vi "初始化.vi"(0 "counter":tag="Dev2/ctr2", 5 "channel name":string="T1", 7 "low time":dbl=0.00026 format="%0.2e", 9 "high time":dbl=0.00024 format="%0.2e", 11 "error in":errorcluster caption="错误输入") -> (4 "task out":refnum<k21> caption="任务输出", 15 "error out":errorcluster caption="错误输出")   [LabVIEW 2020]
uses:
  <vilib>/DAQmx/create/channels.llb/DAQmx Create Channel (CO-Pulse Generation-Time).vi
  <vilib>/DAQmx/configure/timing.llb/DAQmx Timing (Implicit).vi
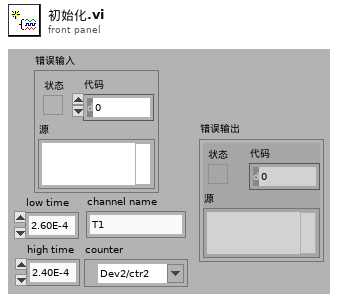
[diagram p1: front panel]
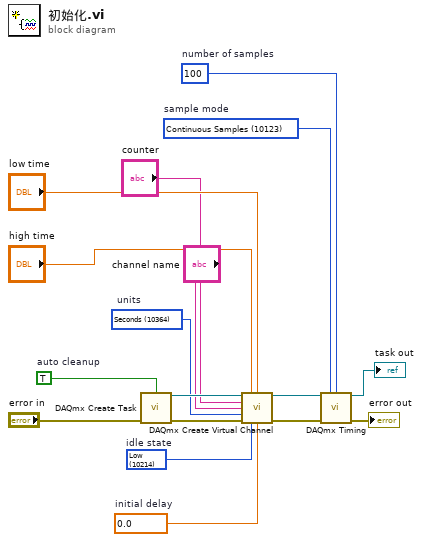
[diagram p0: block diagram]
diagram:
  w2 = 10123 items=["Finite Samples"=10178, "Continuous Samples"=10123, "Hardware Timed Single Point"=12522]  # sample mode
  w3 = 100  # number of samples
  w9 = 0.0  # initial delay
  w10 = 10214 items=["High"=10192, "Low"=10214]  # idle state
  w11 = 10364 items=["Seconds"=10364, "From Custom Scale"=10065]  # units
  w15 = TRUE  # auto cleanup
  n1 = call <vilib>:"DAQmx Create Task.vi"("auto cleanup"=w15, "error in"="error in") -> ("task out"=w14:refnum<k21>, "error out"=w16:errorcluster)  [unwired: 12 in]
  n2 = call-poly <vilib>:"DAQmx Create Virtual Channel.vi"("task in"=w14, "high time"="high time", "low time"="low time", "counter"="counter", "name to assign"="channel name", "units"=w11, "error in"=w16, "idle state"=w10, "initial delay"=w9) -> ("task out"=w4:refnum<k21>, "error out"=w13:errorcluster)  [unwired: 5 in]
  n3 = call-poly <vilib>:"DAQmx Timing.vi"("task/channels in"=w4, "sample mode"=w2, "samples per channel"=w3, "error in"=w13) -> ("task out"=→"task out":refnum<k21>, "error out"=→"error out":errorcluster)  [unwired: 10 in]
